vi "IF2_Reader.vi"(10 "Stop":bool, 11 "RFID Configuration":T1) -> (0 "error out":errorcluster, 3 "connection ID":refnum<k5>)   [LabVIEW 2015, in "IF2_Reader.lvlib"]
uses:
  IF2_Reader.lvlib
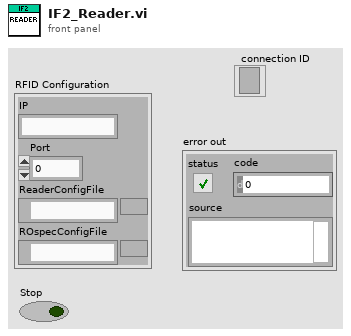
[diagram p1: front panel]
types:
  T1 = cluster{"IP":string, "Port":u16, "ReaderConfigFile":path, "ROspecConfigFile":path}
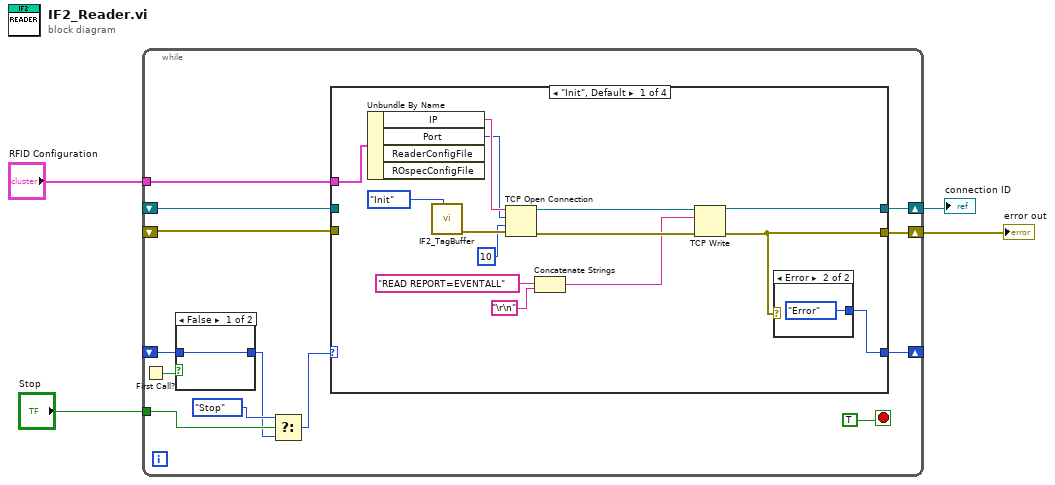
[diagram p0: block diagram]
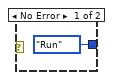
[diagram p2: hidden frame]
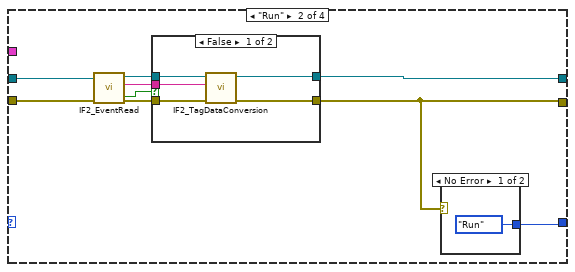
[diagram p3: hidden frame]
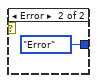
[diagram p5: hidden frame]
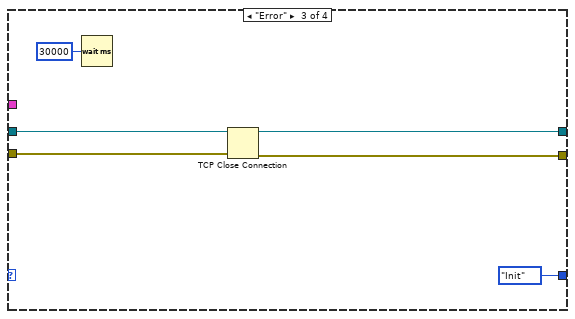
[diagram p6: hidden frame]
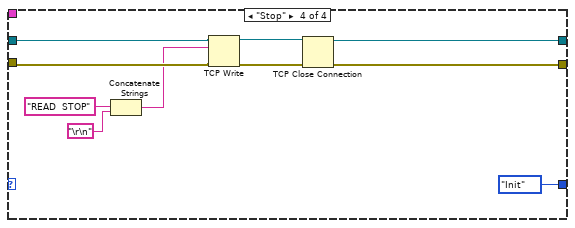
[diagram p7: hidden frame]
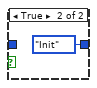
[diagram p8: hidden frame]
diagram:
  n1 = while {
    shift-right: [w7] -> _
    shift-left: _ -> [w15]
    tunnel: "RFID Configuration" -> [w14]
    shift-right: [w13] -> w1
    shift-left: _ -> [w11]
    shift-right: [w12] -> w4
    shift-left: _ -> [w10]
    tunnel: "Stop" -> [w9]
    stop <- TRUE stop-if-true
    n2 = First Call?() -> (First Call?: T/F=w17:bool)
    n3 = case shown="False" w17 {
      tunnel: [w68 enum16{"Stop", "Error", "Run", "Init"}."Init"] -> w5
      tunnel: w15 -> [w68 _]
      frame False {
      }
      frame True {
      }
    }
    n4 = Select(t=enum16{"Stop", "Error", "Run", "Init"}."Stop", s=w9, f=w5) -> (s? t:f=w6:enum16{"Stop", "Error", "Run", "Init"})
    n5 = case shown="\"Init\", Default" w6 {
      tunnel: [w28 w40 enum16{"Stop", "Error", "Run", "Init"}."Init" enum16{"Stop", "Error", "Run", "Init"}."Init"] -> w7
      tunnel: w14 -> [w31 _ _ _]
      tunnel: [w22 w34 w55 w65] -> w13
      tunnel: [w23 w35 w54 w67] -> w12
      tunnel: w11 -> [_ w42 w53 w59]
      tunnel: w10 -> [_ w41 w52 w60]
      frame "Init", Default {
        n6 = Unbundle By Name(w31) -> ("IP"=w30:string, "Port"=w29:u16)  [unwired: 2 out]
        n7 = call "IF2_TagBuffer.vi"("Action"=enum16{"Init", "WriteTagData", "ReadTagData"}."Init") -> ("error out"=w27:errorcluster)  [unwired: 9 in, 1 out]
        n8 = TCP Open Connection(address=w30, remote port or service name=w29, timeout ms (60000)=10, error in (no error)=w27) -> (connection ID=w25:refnum<k5>, error out=w24:errorcluster)  [unwired: 1 in]
        n9 = Concatenate Strings("READ REPORT=EVENTALL" ("data in"), "\r\n") -> (w19:string)
        n10 = TCP Write(connection ID=w25, data in=w19, error in (no error)=w24) -> (connection ID out=w22:refnum<k5>, error out=w23:errorcluster)  [unwired: 2 out]
        n11 = case shown="Error" w23 {
          tunnel: [enum16{"Stop", "Error", "Run", "Init"}."Run" enum16{"Stop", "Error", "Run", "Init"}."Error"] -> w28
          frame No Error {
          }
          frame Error {
          }
        }
      }
      frame "Run" {
        n12 = call "IF2_EventRead.vi"("error in (no error)"=w41, "TCP Network Connection in"=w42) -> ("error out"=w39:errorcluster, "data out"=w37:string, "TCP Network Connection out"=w38:refnum<k5>, "Timeout"=w36:bool)  [unwired: 6 in]
        n13 = case shown="False" w36 {
          tunnel: w39 -> [w47 w48]
          tunnel: w38 -> [w46 w49]
          tunnel: w37 -> [w45 _]
          tunnel: [w43 w48] -> w35
          tunnel: [w44 w49] -> w34
          frame False {
            n14 = call "IF2_TagDataConversion.vi"("error in (no error)"=w47, "IF2 Data"=w45, "TCP Network Connection in"=w46) -> ("error out"=w43:errorcluster, "TCP Network Connection out"=w44:refnum<k5>)  [unwired: 7 in]
          }
          frame True {
          }
        }
        n15 = case shown="No Error" w35 {
          tunnel: [enum16{"Stop", "Error", "Run", "Init"}."Run" enum16{"Stop", "Error", "Run", "Init"}."Error"] -> w40
          frame No Error {
          }
          frame Error {
          }
        }
      }
      frame "Error" {
        n16 = Wait (ms)(milliseconds to wait=u32 30000) -> ()  [unwired: 1 out]
        n17 = TCP Close Connection(connection ID=w53, error in (no error)=w52) -> (connection ID out=w55:refnum<k5>, error out=w54:errorcluster)  [unwired: 1 in]
      }
      frame "Stop" {
        n18 = Concatenate Strings("READ  STOP" ("data in"), "\r\n") -> (w58:string)
        n19 = TCP Write(connection ID=w59, data in=w58, error in (no error)=w60) -> (connection ID out=w62:refnum<k5>, error out=w61:errorcluster)  [unwired: 2 out]
        n20 = TCP Close Connection(connection ID=w62, error in (no error)=w61) -> (connection ID out=w65:refnum<k5>, error out=w67:errorcluster)  [unwired: 1 in]
      }
    }
  }
  "error out" <- w4
  "connection ID" <- w1
